vi "SubVI Logica Pulsos.vi"(7 "Cluster Diferencia de Voltajes":T1, 10 "fase-fase 2":fxp<+/-,17,3>, 11 "fase-fase 1":fxp<+/-,17,3>) -> (0 "Segundo Pulso Negativo":bool, 1 "Primer Pulso Negativo":bool, 2 "Segundo Pulso Positivo":bool, 3 "Primer Pulso Positivo":bool)   [LabVIEW 2020]
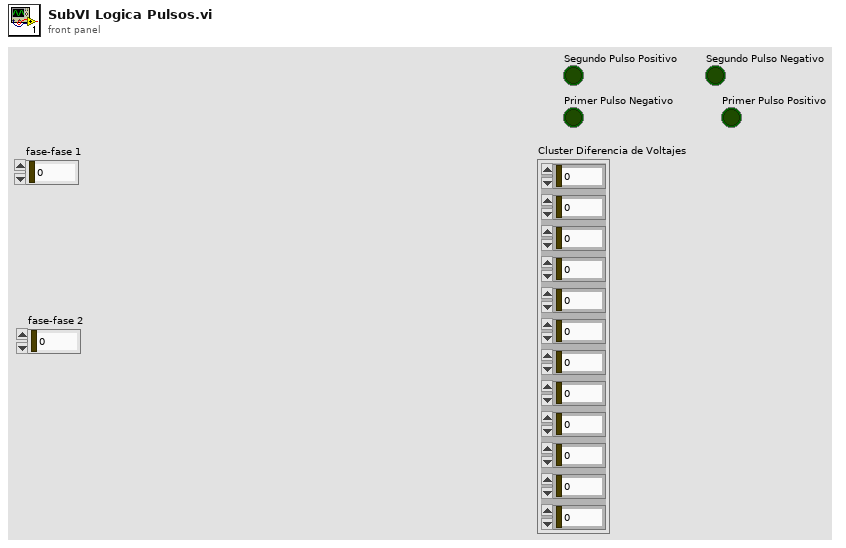
[diagram p1: front panel]
types:
  T1 = cluster{fxp<+/-,17,3>, fxp<+/-,17,3>, fxp<+/-,17,3>, fxp<+/-,17,3>, fxp<+/-,17,3>, fxp<+/-,17,3>, fxp<+/-,17,3>, fxp<+/-,17,3>, fxp<+/-,17,3>, fxp<+/-,17,3>, fxp<+/-,17,3>, fxp<+/-,17,3>}
  T2 = cluster{fxp<+,16,2>, fxp<+,16,2>, fxp<+,16,2>, fxp<+,16,2>, fxp<+,16,2>, fxp<+,16,2>, fxp<+,16,2>, fxp<+,16,2>, fxp<+,16,2>, fxp<+,16,2>, fxp<+,16,2>, fxp<+,16,2>}
  T3 = cluster{bool, bool, bool, bool, bool, bool, bool, bool, bool, bool, bool, bool}
  T4 = cluster{fxp<+/-,33,5>, fxp<+/-,33,5>, fxp<+/-,33,5>, fxp<+/-,33,5>, fxp<+/-,33,5>, fxp<+/-,33,5>, fxp<+/-,33,5>, fxp<+/-,33,5>, fxp<+/-,33,5>, fxp<+/-,33,5>, fxp<+/-,33,5>, fxp<+/-,33,5>}
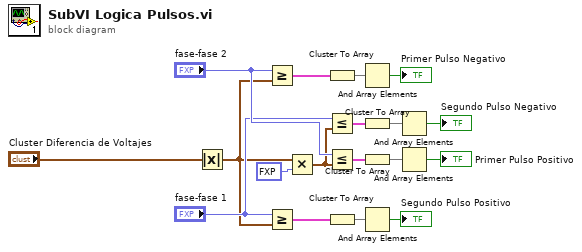
[diagram p0: block diagram]
diagram:
  n1 = Absolute Value(x="Cluster Diferencia de Voltajes") -> (abs(x)=w2:T2)
  n2 = Greater Or Equal?(x="fase-fase 2", y=w2) -> (x >= y?=w14:T3)
  n3 = Greater Or Equal?(x="fase-fase 1", y=w2) -> (x >= y?=w16:T3)
  n4 = Multiply(x=w2, y=fxp<+/-,17,3> -1.0 ("DOWN 4")) -> (x*y=w1:T4)
  n5 = Cluster To Array(cluster=w14) -> (array=w12:bool[])
  n6 = Less Or Equal?(x="fase-fase 1", y=w1) -> (x <= y?=w15:T3)
  n7 = Less Or Equal?(x="fase-fase 2", y=w1) -> (x <= y?=w4:T3)
  n8 = Cluster To Array(cluster=w16) -> (array=w7:bool[])
  n9 = And Array Elements(Boolean array=w12) -> (logical AND=→"Primer Pulso Negativo":bool)
  n10 = Cluster To Array(cluster=w15) -> (array=w17:bool[])
  n11 = Cluster To Array(cluster=w4) -> (array=w3:bool[])
  n12 = And Array Elements(Boolean array=w7) -> (logical AND=→"Segundo Pulso Positivo":bool)
  n13 = And Array Elements(Boolean array=w17) -> (logical AND=→"Segundo Pulso Negativo":bool)
  n14 = And Array Elements(Boolean array=w3) -> (logical AND=→"Primer Pulso Positivo":bool)
